vi "Initialize Client IO Test.vi"(10 "channel classification":T4) -> (0 "error out":errorcluster, 1 "OPC UA server refnum out":refnum<k21>, 2 "data allocations":T1, 3 "OPC UA runtime out":refnum<class "OPC UA Client runtime.lvclass">, 4 "Lines":T5[](array[typedef]) {"OPC UA Data Type" items=["Boolean"=1, "SByte"=2, "Byte"=3, "Int16"=4, "UInt16"=5, "Int32"=6, "UInt32"=7, "Int64"=8, "UInt64"=9, "Float"=10, "Double"=11, "String"=12, "DateTime"=13, "ByteString"=15, "Array of Boolean"=101, "Array of SByte"=102, "Array of Byte"=103, "Array of Int16"=104, "Array of UInt16"=105, "Array of Int32"=106, "Array of UInt32"=107, "Array of Int64"=108, "Array of UInt64"=109, "Array of Float"=110, "Array of Double"=111, "Array of String"=112, "Array of DateTime"=113, "Array of ByteString"=115]})   [LabVIEW 2013, in "OPC UA Client Tests.lvlib"]
doc: "Initializes OPC UA test server and client connection for testing input and output overrides."
uses:
  OPC UA Client Tests.lvlib
  module/execution/OPC UA Client runtime.lvclass
  module/configuration/Line.ctl
  <vilib>/NI/Tag Bus Module Framework/channel/TBM channel.lvclass
  module/configuration/OPC UA Data Type.ctl
  <vilib>/NI/Tag Bus Module Framework/channel/channel classification.ctl
  <vilib>/NI/Tag Bus Module Framework/channel/data tables.ctl
  <vilib>/NI/Tag Bus/dictionary/data dictionary.lvclass
  <vilib>/NI/Tag Bus/dictionary table pair.ctl
  <vilib>/NI/Tag Bus/table/data table.ctl
  Server Connection Configuration.ctl
  <vilib>/OPCUA/server/subVI/supported security policies.ctl
  module/configuration/Client Connection Configuration.ctl
  module/configuration/OPC UA Client configuration.lvclass/OPC UA Client configuration.ctl
  module/configuration/Read Lines.vi
  module/configuration/OPC UA Client configuration.lvclass
  <vilib>/opcua/NI OPC UA Server.lvlib
  <vilib>/NI/Tag Bus/table/data table.lvlib
  <vilib>/NI/Tag Bus/tag bus.lvlib
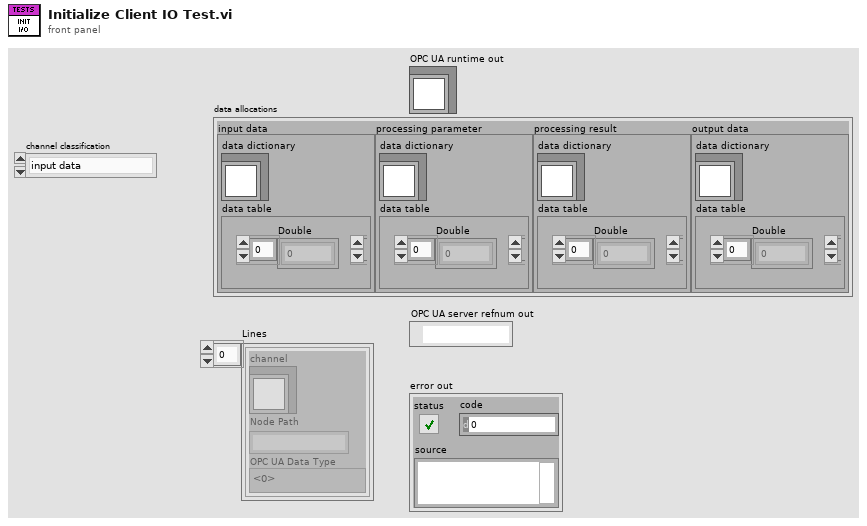
[diagram p1: front panel]
types:
  T1 = typedef "TBM channel.lvclass/data tables.ctl" = cluster{"input data":T2, "processing parameter":T2, "processing result":T2, "output data":T2}
  T2 = typedef "tag bus.lvlib/dictionary table pair.ctl" = cluster{"data dictionary":refnum<class "data dictionary.lvclass">, "data table":T3}
  T3 = typedef "tag bus.lvlib/data table.lvlib/data table.ctl" = cluster{"Double":dbl[], "Single":sgl[], "I64":i64[], "I32":i32[], "I16":i16[], "I8":i8[], "U64":u64[], "U32":u32[], "U16":u16[], "U8":u8[], "Boolean":bool[], "String":string[], "Array of Double":cluster{"DBL Array":dbl[]}[], "Array of Single":cluster{"SGL Array":sgl[]}[], "Array of I64":cluster{"I64 Array":i64[]}[], "Array of I32":cluster{"I32 Array":i32[]}[], "Array of I16":cluster{"I16 Array":i16[]}[], "Array of I8":cluster{"I8 Array":i8[]}[], "Array of U64":cluster{"U64 Array":u64[]}[], "Array of U32":cluster{"U32 Array":u32[]}[], "Array of U16":cluster{"U16 Array":u16[]}[], "Array of U8":cluster{"U8 Array":u8[]}[], "Array of Boolean":cluster{"Boolean Array":bool[]}[], "Array of String":cluster{"String Array":string[]}[]}
  T4 = typedef "TBM channel.lvclass/channel classification.ctl" = enum16{"input data", "output data", "processing parameter", "processing result"}
  T5 = typedef "OPC UA Client configuration.lvclass/Line.ctl" = cluster{"channel":refnum<class "TBM channel.lvclass">, "Node Path":string, "OPC UA Data Type":T6}
  T6 = typedef "OPC UA Client configuration.lvclass/OPC UA Data Type.ctl" = u16
  T7 = typedef "OPC UA Client configuration.lvclass/Client Connection Configuration.ctl" = cluster{"Server Certificates":cluster{"Relative Path?":bool, "Absolute Paths":string[], "Relative Paths":string[]}, "Client Certificates":cluster{"Relative Path?":bool, "Absolute Path":string, "Relative Path":string}, "Client Configuration":cluster{"Server Endpoint URL":string, "Security Policy":cluster{"Message Mode":enum16{"None", "Sign", "Sign and Encrypt"}, "Security":enum16{"Basic256", "Basic128Rsa15"}}, "Username/Password":cluster{"Username":string, "Password":string}}}
  T8 = typedef "OPC UA Client Tests.lvlib/Server Connection Configuration.ctl" = cluster{"Server Certificates":cluster{"Relative Path?":bool, "Certificate Paths":path[], "Certificate Names":string[]}, "Client Certificates":cluster{"Relative Path?":bool, "Certificate Paths":path[], "Certificate Names":string[]}, "Server Configuration":cluster{"Server Name":string, "TCP port (49580)":string, "Supported Security Policies":T9}}
  T9 = typedef "supported security policies.ctl" = cluster{"None":bool, "Sign with Basic128Rsa125":bool, "Sign and Encrypt with Basic128Rsa125":bool, "Sign with Basic256":bool, "Sign and Encrypt with Basic256":bool}
  T10 = typedef "OPC UA configuration.lvclass/Line.ctl" = cluster{"channel":refnum<class "TBM channel.lvclass">, "Node Path":string, "OPC UA Data Type":T11}
  T11 = typedef "OPC UA configuration.lvclass/OPC UA Data Type.ctl" = u16
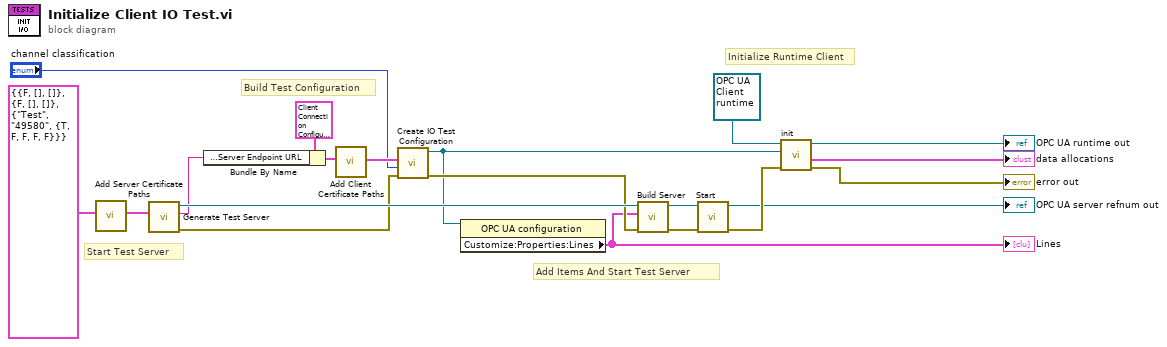
[diagram p0: block diagram]
diagram:
  # "Initialize Runtime Client"
  # "Add Items And Start Test Server"
  # "Start Test Server"
  # "Build Test Configuration"
  n1 = call "Add Server Certificate Paths.vi"("Server Connection Configuration In"=T8 {"Server Certificates"={"Relative Path?"=FALSE, "Certificate Paths"=[], "Certificate Names"=[]}, "Client Certificates"={"Relative Path?"=FALSE, "Certificate Paths"=[], "Certificate Names"=[]}, "Server Configuration"={"Server Name"="Test", "TCP port (49580)"="49580", "Supported Security Policies"={"None"=TRUE, "Sign with Basic128Rsa125"=FALSE, "Sign and Encrypt with Basic128Rsa125"=FALSE, "Sign with Basic256"=FALSE, "Sign and Encrypt with Basic256"=FALSE}}} ("Server Connection Configuration")) -> ("Server Connection Configuration Out"=w10:T8)  [unwired: 10 in]
  n2 = call "Generate Test Server.vi"("Server Connection Configuration"=w10) -> ("OPC UA server refnum out"=w18:refnum<k21>, "server endpoint URL"=w13:string, "error out"=w7:errorcluster)  [unwired: 7 in]
  n3 = Bundle By Name(cluster=T7 {"Server Certificates"={"Relative Path?"=FALSE, "Absolute Paths"=[], "Relative Paths"=[]}, "Client Certificates"={"Relative Path?"=FALSE, "Absolute Path"="", "Relative Path"=""}, "Client Configuration"={"Server Endpoint URL"="", "Security Policy"={"Message Mode"=enum."None", "Security"=enum."Basic256"}, "Username/Password"={"Username"="", "Password"=""}}} ("Client Connection Configuration"), "Client Configuration.Server Endpoint URL"=w13) -> (w11:T7)
  n4 = call "Add Client Certificate Paths.vi"("Client Connection Configuration In"=w11) -> ("Client Connection Configuration Out"=w4:T7)  [unwired: 10 in]
  n5 = call "Create IO Test Configuration.vi"("Error In"=w7, "channel classification"="channel classification", "Client Connection Configuration"=w4) -> ("Error Out"=w6:errorcluster, "module"=w5:refnum<class "OPC UA Client configuration.lvclass">)  [unwired: 7 in]
  n6 = property class="OPC UA configuration"(reference=w5) -> ("Customize:Properties:Lines"=w3:T10[])  [unwired: 1 in, 2 out]
  "Lines" <- w3
  n7 = call "Build Server.vi"("Error In"=w6, "Lines"=w3, "OPC UA server refnum in"=w18) -> ("Error Out"=w17:errorcluster, "OPC UA server refnum out"=w15:refnum<k21>)  [unwired: 7 in]
  n8 = call <vilib>:"Start.vi"("error in (no error)"=w17, "OPC UA server refnum in"=w15) -> ("error out"=w16:errorcluster, "OPC UA server refnum out"=→"OPC UA server refnum out":refnum<k21>)  [unwired: 8 in]
  n9 = call-dynamic "init.vi"("error in"=w16, "TBM module configuration in"=w5, "OPC UA runtime in"=refnum<class "OPC UA Client runtime.lvclass"> refnum ("OPC UA runtime")) -> ("error out"=→"error out":errorcluster, "data allocations"=→"data allocations":T1, "OPC UA runtime out"=→"OPC UA runtime out":refnum<class "OPC UA Client runtime.lvclass">)  [unwired: 5 in, 1 out]
